vi "Create Engine Simulation Toolkit Custom Device.vi"(8 "error in (no error)":errorcluster, 10 "Engine Simulation Toolkit Custom Device Settings":T1={"Name"="", "Execution priority"=enum."Low", "Rate decimation"=1, "CPU"=-2, "Device address"="RIO 0", "Bitfile path"=path "", "APUs"=[]}, 11 "Target in":refnum<k24>) -> (0 "error out":errorcluster, 2 "EST Custom Device":refnum<k24>, 3 "Target out":refnum<k24>)   [LabVIEW 2015, in "Engine Simulation Toolkit SysDef API.lvlib"]
uses:
  Engine Simulation Toolkit SysDef API.lvlib
  NationalInstruments.VeriStand.SystemDefinitionAPI
  Engine Simulation Toolkit Custom Device Settings.ctl
  <vilib>/NI Veristand/Custom Device API/Custom Device Timed Loop Priority.ctl
  <vilib>/NI Veristand/Custom Device API/Dependent File Optional Info.ctl
  Shared/Constants and GUIDs.vi
  Shared/Properties.vi
  <vilib>/NI/NI VeriStand Advanced SysDef API/_SubVIs/SysDef.Property.Set.I32.vi
  <vilib>/NI/NI VeriStand Advanced SysDef API/_SubVIs/SysDef.Property.Set.String.vi
  System Explorer/Engine Simulation Toolkit System Explorer.lvlib
  Shared/Engine Simulation Toolkit Shared.lvlib
  <vilib>/NI Veristand/Custom Device API/Custom Device API.lvlib
  <vilib>/NI/NI VeriStand Advanced SysDef API/SysDef API/Advanced System Definition.lvlib
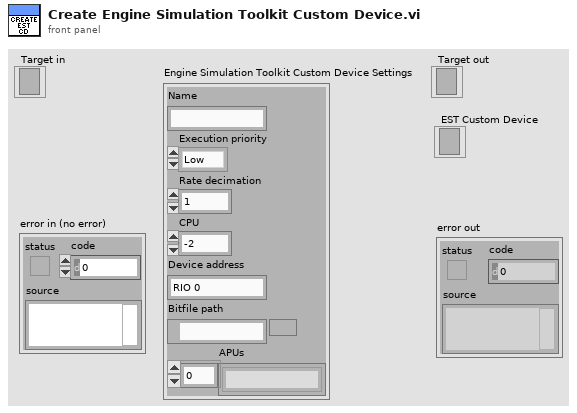
[diagram p1: front panel]
types:
  T1 = typedef "Engine Simulation Toolkit SysDef API.lvlib/Engine Simulation Toolkit Custom Device Settings.ctl" = cluster{"Name":string, "Execution priority":T2, "Rate decimation":i32, "CPU":i32, "Device address":string, "Bitfile path":path, "APUs":string[]}
  T2 = typedef "Custom Device API.lvlib/Custom Device Timed Loop Priority.ctl" = enum32{"Low", "Medium", "High"}
  T3 = typedef "Custom Device API.lvlib/Dependent File Optional Info.ctl" = cluster{"Version":string, "RTDestination":path, "ForceDownload":bool, "SupportedTarget":string, "MD5":string}
  T4 = typedef "Custom Device API.lvlib/Custom Device Item Ref.ctl" = u64
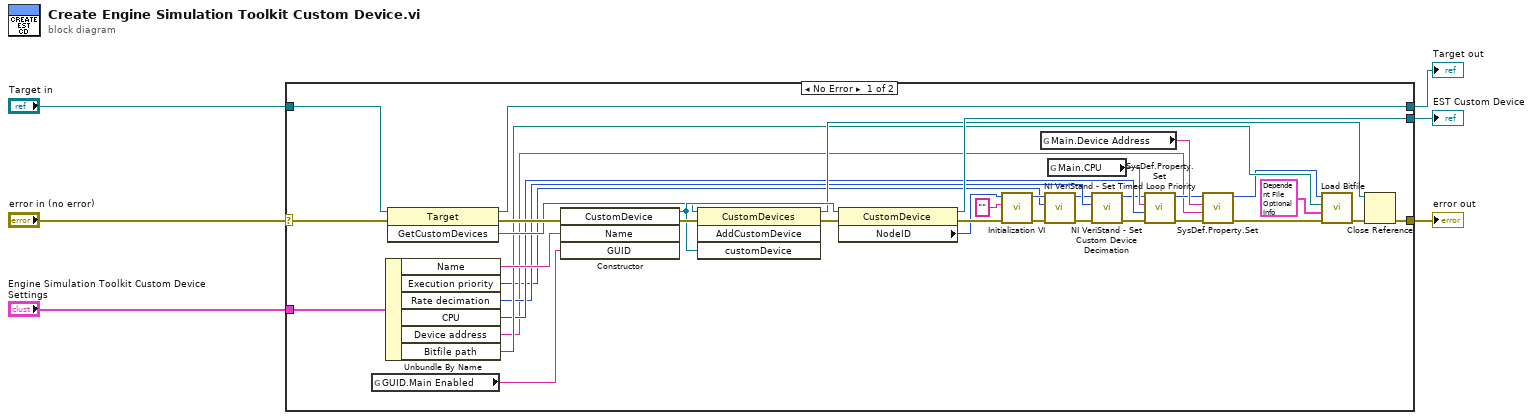
[diagram p0: block diagram]
diagram:
  n1 = case shown="No Error" "error in (no error)" {
    selector: "error in (no error)" -> [w42 w44]
    tunnel: [w25 w44] -> w6
    tunnel: "Target in" -> [w37 w43]
    tunnel: [w41 w43] -> w3
    tunnel: "Engine Simulation Toolkit Custom Device Settings" -> [w34 _]
    tunnel: [w30 _] -> w1
    frame No Error {
      n2 = global read "Constants and GUIDs.vi" "GUID.Main Enabled"() -> (w32:string)
      n3 = Unbundle By Name(w34) -> ("Name"=w33:string, "Execution priority"=w7:T2, "Rate decimation"=w18:i32, "CPU"=w19:i32, "Device address"=w8:string, "Bitfile path"=w23:path)
      n4 = invoke class="Target" method="GetCustomDevices"(reference=w37, error in=w42) -> (reference out=w41:refnum<k24>, error out=w36:errorcluster, "GetCustomDevices"=w28:refnum<k24>)  [unwired: 1 in]
      n5 = constructor class="CustomDevice"(error in=w36, "Name"=w33, "GUID"=w32) -> (reference out=w31:refnum<k24>, error out=w39:errorcluster)  [unwired: 2 in, 3 out]
      n6 = invoke class="CustomDevices" method="AddCustomDevice"(reference=w28, error in=w39, "customDevice"=w31) -> (reference out=w24:refnum<k24>, error out=w40:errorcluster)  [unwired: 1 in, 2 out]
      n7 = property class="CustomDevice"(reference=w31, error in=w40) -> (reference out=w30:refnum<k24>, error out=w38:errorcluster, "NodeID"=w29:u64)
      n8 = call "Initialization VI.vi"("error in (no error)"=w38, "Custom XML"="", "Device Item Ref in"=w29) -> ("error out"=w20:errorcluster, "Device Item Ref out"=w21:T4)  [unwired: 7 in]
      n9 = global read "Properties.vi" "Main.Device Address"() -> (w13:string)
      n10 = call <vilib>:"NI VeriStand - Set Timed Loop Priority.vi"("error in (no error)"=w20, "Priority"=w7, "Device Ref in"=w21) -> ("error out"=w17:errorcluster, "Device Ref out"=w15:T4)  [unwired: 7 in]
      n11 = global read "Properties.vi" "Main.CPU"() -> (w22:string)
      n12 = call <vilib>:"NI VeriStand - Set Custom Device Decimation.vi"("error in (no error)"=w17, "Decimation"=w18, "Device Ref in"=w15) -> ("error out"=w16:errorcluster, "Device Ref out"=w14:T4)  [unwired: 7 in]
      n13 = call-poly <vilib>:"SysDef.Property.Set.vi"("error in (no error)"=w16, "Value"=w19, "Property Name"=w22, "nodeID"=w14) -> ("error out"=w10:errorcluster, "nodeID out"=w12:u64)  [unwired: 6 in]
      n14 = call-poly <vilib>:"SysDef.Property.Set.vi"("error in (no error)"=w10, "Value"=w8, "Property Name"=w13, "nodeID"=w12) -> ("error out"=w9:errorcluster, "nodeID out"=w11:u64)  [unwired: 6 in]
      n15 = call "Load Bitfile.vi"("error in (no error)"=w9, "OptionalInfo"=T3 {"Version"="1.0", "RTDestination"=path "c:/ni-rt/NIVeriStand/Custom Devices/Engine Simulation Toolkit", "ForceDownload"=FALSE, "SupportedTarget"="All", "MD5"=""}, "NewVal"=w23, "Section Ref in"=w11) -> ("error out"=w26:errorcluster)  [unwired: 5 in, 2 out]
      n16 = Close Reference(reference=w24, error in (no error)=w26) -> (error out=w25:errorcluster)
    }
    frame Error {
    }
  }
  "error out" <- w6
  "Target out" <- w3
  "EST Custom Device" <- w1
